vi "get_speed_by_name.vi"(8 "error in (no error)":errorcluster caption="错误输入（无错误）", 10 "String":string, 11 "MotorSystem 输入":refnum<class "MotorSystem.lvclass">) -> (0 "error out":errorcluster caption="错误输出", 2 "speed":i32, 3 "MotorSystem 输出":refnum<class "MotorSystem.lvclass">)   [LabVIEW 2016, in "MotionControl_UFO_3DOF.lvlib" / "MotorSystem.lvclass"]
uses:
  <userlib>/MotionControl_UFO_3DOF/MotorSystem/MotorSystem.lvclass
  <userlib>/MotionControl_UFO_3DOF/MotorSystem/MotorSystem.lvclass/MotorSystem.ctl
  <userlib>/MotionControl_UFO_3DOF/OneMotion/OneMotion.lvclass
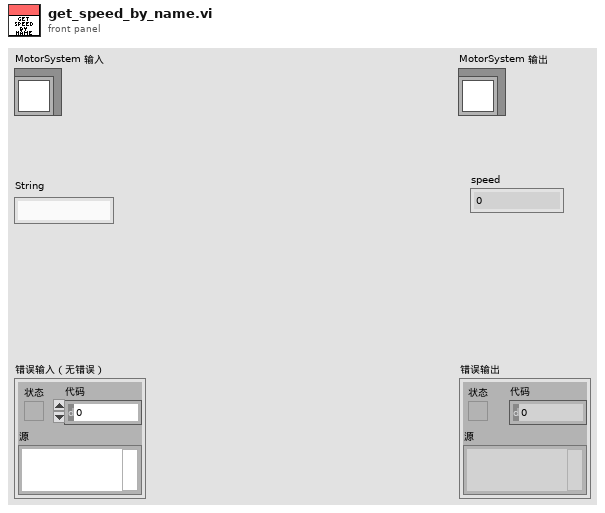
[diagram p1: front panel]
types:
  T1 = typedef "MotionControl_UFO_3DOF.lvlib/MotorSystem.lvclass/MotionCluster.ctl" = cluster{"OneMotion.lvclass":refnum<class "OneMotion.lvclass">, "connected?":bool, "default enabled?":bool, "enabled?":bool}
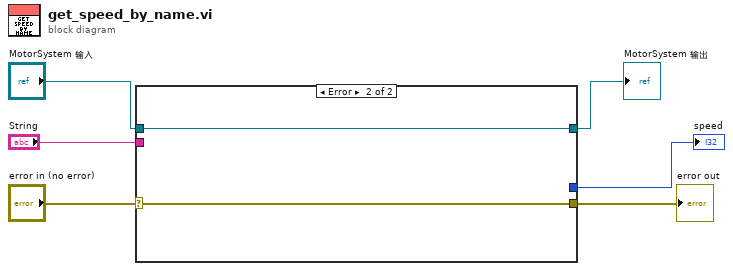
[diagram p0: block diagram]
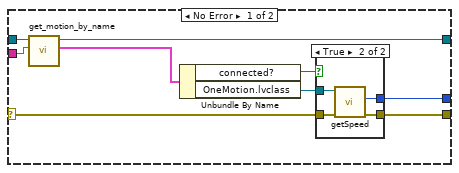
[diagram p2: hidden frame]
diagram:
  n1 = case shown="Error" "error in (no error)" {
    selector: "error in (no error)" -> [w15 w22]
    tunnel: [w14 w22] -> w5
    tunnel: [w12 w21] -> w3
    tunnel: "MotorSystem 输入" -> [w11 w21]
    tunnel: "String" -> [w10 _]
    tunnel: [w9 _] -> w1
    frame No Error {
      n2 = call <userlib>:"get_motion_by_name.vi"("name"=w10, "MotorSystem in"=w11) -> ("motion cluster"=w8:T1, "MotorSystem out"=w12:refnum<class "MotorSystem.lvclass">)  [unwired: 7 in, 1 out]
      n3 = Unbundle By Name(w8) -> ("connected?"=w13:bool, "OneMotion.lvclass"=w7:refnum<class "OneMotion.lvclass">)
      n4 = case shown="True" w13 {
        tunnel: w15 -> [w16 w20]
        tunnel: [w16 w19] -> w14
        tunnel: [_ w18] -> w9
        tunnel: w7 -> [_ w17]
        frame False {
        }
        frame True {
          n5 = call <userlib>:"getSpeed.vi"("error in (no error)"=w20, "OneMotion 输入"=w17) -> ("error out"=w19:errorcluster, "speed"=w18:i32)  [unwired: 7 in, 1 out]
        }
      }
    }
    frame Error {
    }
  }
  "error out" <- w5
  "MotorSystem 输出" <- w3
  "speed" <- w1
